vi "Port.vi"(8 "error in (no error)":errorcluster, 11 "Node Ptr":T1 format="%.0x") -> (0 "error out":errorcluster)   [LabVIEW 2020, in "Communication Bus Template System Explorer.lvlib" / "Implementation.lvlib"]
uses:
  Implementation.lvlib
  <vilib>/NI VeriStand/Custom Device API/Custom Device Item Ref.ctl
  <vilib>/NI VeriStand/Custom Device API/Custom Device API.lvlib
  Scripting/Communication Bus Template Scripting.lvlib
panel:
  in  "Baud Rate":u32
  in  "Database":string(combo)
  in  "SHDocVw.IWebBrowser":refnum<k7>(container)
  in  "Specific Header":cluster{"Section Name":string}={"Section Name"="Specific Page Settings"}
  in  "General Header":cluster{"Section Name":string}={"Section Name"="General Page Settings"}
  in  "Description":string
  in  "Name":string
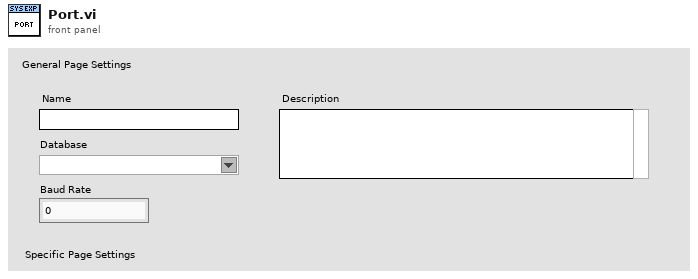
[diagram p1: front panel]
types:
  T1 = typedef "Custom Device API.lvlib/Custom Device Item Ref.ctl" = u64
  T2 = typedef "Custom Device API.lvlib/Custom Device Item Info.ctl" = cluster{"Name":string, "Is Channel":bool, "GUID":string, "Is Waveform":bool}
  T3 = typedef "Custom Device API.lvlib/Custom Device Commands.ctl" = enum16{"Default", "Item renamed", "Shutdown", "Dynamic button pressed"}
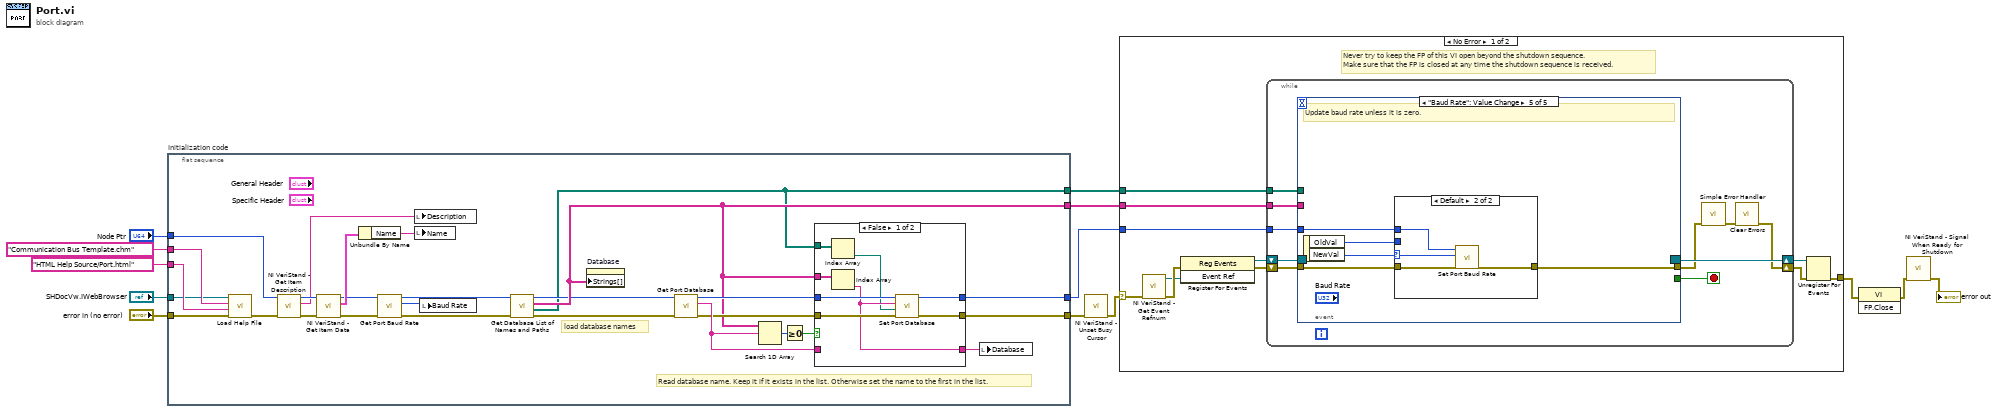
[diagram p0: block diagram]
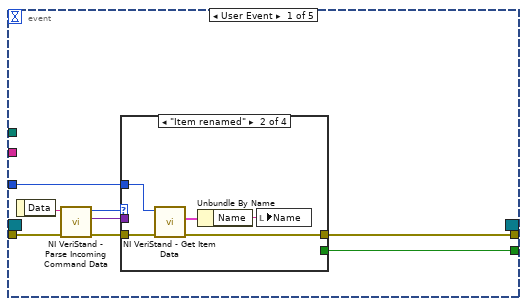
[diagram p3: hidden frame]
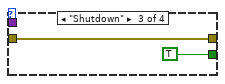
[diagram p5: hidden frame]
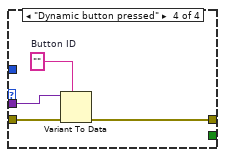
[diagram p6: hidden frame]
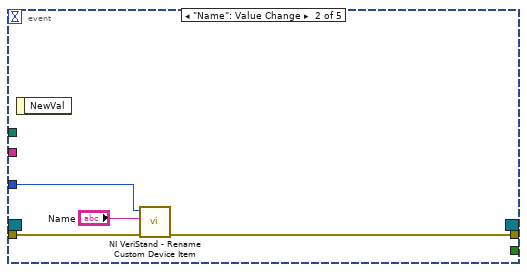
[diagram p7: hidden frame]
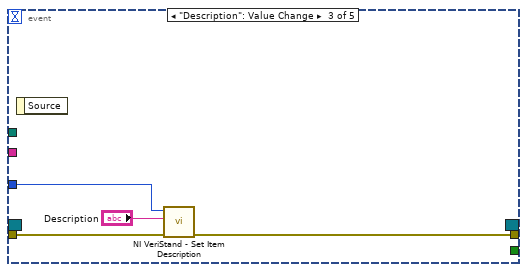
[diagram p8: hidden frame]
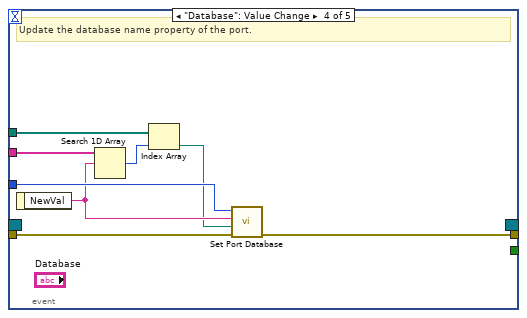
[diagram p9: hidden frame]
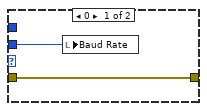
[diagram p10: hidden frame]
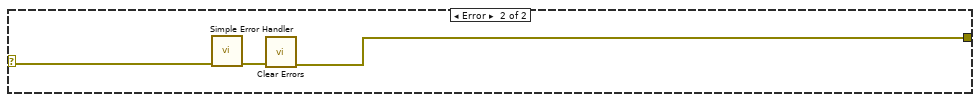
[diagram p11: hidden frame]
diagram:
  n1 = flat-sequence "Initialization code" {
    tunnel: "error in (no error)" -> [w35]
    tunnel: "Node Ptr" -> [w38]
    tunnel: [w30] -> w9
    tunnel: [w29] -> w6
    tunnel: "SHDocVw.IWebBrowser" -> [w31]
    tunnel: "HTML Help Source/Port.html" ("CD_CHM_Section") -> [w33]
    tunnel: "Communication Bus Template.chm" ("CD_CHM_FileName") -> [w32]
    tunnel: [w14] -> w2
    tunnel: [w18] -> w1
    frame #0 {
      # "Read database name. Keep it if it exists in the list. Otherwise set the name to the first in the list."
      # "load database names"
      n2 = call "Load Help File.vi"("error in (no error)"=w35, "HTML File to Load"=w33, "Main CHM File"=w32, "Browser"=w31) -> ("error out"=w34:errorcluster)  [unwired: 7 in]
      n3 = call <vilib>:"NI VeriStand - Get Item Description.vi"("error in (no error)"=w34, "Item Ref in"=w38) -> ("error out"=w40:errorcluster, "Description"=w36:string, "Item Ref out"=w41:T1)  [unwired: 7 out]
      n4 = call <vilib>:"NI VeriStand - Get Item Data.vi"("error in (no error)"=w40, "Item Ref in"=w41) -> ("error out"=w22:errorcluster, "Item Info"=w39:T2, "Item Ref out"=w21:T1)  [unwired: 7 out]
      n5 = Unbundle By Name(w39) -> ("Name"=w37:string)
      n6 = call "Get Port Baud Rate.vi"("error in"=w22, "Port Ref"=w21) -> ("error out"=w19:errorcluster, "Baud Rate"=w23:u32, "Port Ref out"=w20:T1)  [unwired: 7 in]
      n7 = local write "Description"(w36) -> ()
      n8 = local write "Name"(w37) -> ()
      n9 = local write "Baud Rate"(w23) -> ()
      n10 = call "Get Database List of Names and Paths.vi"("error in"=w19, "Databases section Ref"=w20) -> ("error out"=w16:errorcluster, "Paths"=w14:path[], "Names"=w18:string[], "Databases section Ref out"=w17:T1)  [unwired: 6 in]
      n11 = property on="Database" class="CmbBox"("Strings[]"=w18) -> ()  [unwired: 2 in, 2 out]
      n12 = call "Get Port Database.vi"("error in"=w16, "Port Ref"=w17) -> ("error out"=w24:errorcluster, "Database Name"=w25:string, "Port Ref out"=w28:T1)  [unwired: 5 in, 2 out]
      n13 = Search 1D Array(1D array=w18, element=w25) -> (index of element=w15:i32)  [unwired: 1 in]
      n14 = Greater Or Equal To 0?(x=w15) -> (x >= 0?=w27:bool)
      n15 = case shown="False" w27 {
        tunnel: [w46 w51] -> w30
        tunnel: [w47 w52] -> w29
        tunnel: w24 -> [w45 w51]
        tunnel: w28 -> [w48 w52]
        tunnel: [w44 w50] -> w26
        tunnel: w25 -> [_ w50]
        tunnel: w18 -> [w49 _]
        tunnel: w14 -> [w43 _]
        frame False {
          n16 = Index Array(array=w43) -> (element=w42:path)  [unwired: 1 in]
          n17 = Index Array(array=w49) -> (element=w44:string)  [unwired: 1 in]
          n18 = call "Set Port Database.vi"("error in"=w45, "Database Path"=w42, "Database Name"=w44, "Port Ref"=w48) -> ("error out"=w46:errorcluster, "Port Ref out"=w47:T1)  [unwired: 6 in]
        }
        frame True {
        }
      }
      n19 = local write "Database"(w26) -> ()
    }
  }
  n20 = call <vilib>:"NI VeriStand - Unset Busy Cursor.vi"("error in (no error)"=w9) -> ("error out"=w8:errorcluster)  [unwired: 10 out]
  n21 = case shown="No Error" w8 {
    selector: w8 -> [w55 w123]
    tunnel: [w60 w121] -> w13
    tunnel: w6 -> [w56 _]
    tunnel: w2 -> [w54 _]
    tunnel: w1 -> [w53 _]
    frame No Error {
      # "Never try to keep the FP of this VI open beyond the shutdown sequence.\nMake sure that the FP is closed at any time the shutdown sequence is received."
      n22 = call <vilib>:"NI VeriStand - Get Event Refnum.vi"("error in (no error)"=w55) -> ("error out"=w63:errorcluster, "Event Ref"=w59:refnum<user-event>)  [unwired: 9 out]
      n23 = register-events(error in=w63, w59) -> (reference out=w57:refnum<event-registration>, error out=w58:errorcluster)  [unwired: 1 in]
      n24 = while {
        tunnel: w56 -> [w69]
        shift-right: [w66] -> w61
        shift-left: w58 -> [w72]
        shift-right: [w73] -> w62
        shift-left: w57 -> [w71]
        tunnel: w54 -> [w65]
        tunnel: w53 -> [w64]
        stop <- w70 stop-if-true
        n25 = event shown="[4] \"Baud Rate\": Value Change" {
          selector: w71 -> [_ _ _ _ _]
          dyn-events: [_ _ _ _ _] -> w73
          timeout: _ -> [_ _ _ _ _]
          tunnel: w72 -> [w81 w97 w100 w109 w114]
          tunnel: [w77 _ _ _ _] -> w70
          tunnel: [w76 w96 w99 w105 w112] -> w68
          tunnel: w69 -> [w75 w95 w101 w104 w111]
          tunnel: w65 -> [_ _ _ w108 _]
          tunnel: w64 -> [_ _ _ w107 _]
          event User Event {
            n26 = event-data() -> ("Data"=w80:string)  [unwired: 1 out]
            n27 = call <vilib>:"NI VeriStand - Parse Incoming Command Data.vi"("error in (no error)"=w81, "Incoming data"=w80) -> ("error out"=w79:errorcluster, "Outgoing data"=w74:variant, "Action"=w78:T3)  [unwired: 7 out]
            n28 = case shown="\"Item renamed\"" w78 {
              tunnel: w79 -> [w82 w87 w88 w93]
              tunnel: [_ _ TRUE _] -> w77
              tunnel: [w82 w84 w88 w90] -> w76
              tunnel: w75 -> [_ w86 _ _]
              tunnel: w74 -> [_ _ _ w92]
              frame "Default", Default {
              }
              frame "Item renamed" {
                n29 = call <vilib>:"NI VeriStand - Get Item Data.vi"("error in (no error)"=w87, "Item Ref in"=w86) -> ("error out"=w84:errorcluster, "Item Info"=w85:T2)  [unwired: 8 out]
                n30 = Unbundle By Name(w85) -> ("Name"=w83:string)
                n31 = local write "Name"(w83) -> ()
              }
              frame "Shutdown" {
              }
              frame "Dynamic button pressed" {
                w91 = ""  # Button ID
                n32 = Variant To Data(error in=w93, type=w91, Variant=w92) -> (error out=w90:errorcluster)  [unwired: 1 out]
              }
            }
          }
          event "Name": Value Change {
            n33 = event-data() -> ()  [unwired: 2 out]
            n34 = call <vilib>:"NI VeriStand - Rename Custom Device Item.vi"("error in (no error)"=w97, "New Name"="Name", "Item Ref in"=w95) -> ("error out"=w96:errorcluster)  [unwired: 1 in, 7 out]
          }
          event "Description": Value Change {
            n35 = event-data() -> ()  [unwired: 2 out]
            n36 = call <vilib>:"NI VeriStand - Set Item Description.vi"("error in (no error)"=w100, "Description"="Description", "Item Ref in"=w101) -> ("error out"=w99:errorcluster)  [unwired: 8 out]
          }
          event "Database": Value Change {
            # "Update the database name property of the port."
            n37 = event-data() -> ("NewVal"=w103:string)  [unwired: 1 out]
            n38 = Search 1D Array(1D array=w107, element=w103) -> (index of element=w106:i32)  [unwired: 1 in]
            n39 = Index Array(array=w108, index=w106) -> (element=w102:path)
            n40 = call "Set Port Database.vi"("error in"=w109, "Database Path"=w102, "Database Name"=w103, "Port Ref"=w104) -> ("error out"=w105:errorcluster)  [unwired: 6 in, 1 out]
          }
          event "Baud Rate": Value Change {
            # "Update baud rate unless it is zero."
            n41 = event-data() -> ("OldVal"=w110:u32, "NewVal"=w113:u32)  [unwired: 1 out]
            n42 = case shown="Default" w113 {
              selector: w113 -> [_ w117]
              tunnel: w114 -> [w116 w120]
              tunnel: [w116 w119] -> w112
              tunnel: w111 -> [_ w118]
              tunnel: w110 -> [w115 _]
              frame 0 {
                n43 = local write "Baud Rate"(w115) -> ()
              }
              frame Default {
                n44 = call "Set Port Baud Rate.vi"("error in"=w120, "Baud Rate"=w117, "Port Ref"=w118) -> ("error out"=w119:errorcluster)  [unwired: 7 in, 1 out]
              }
            }
          }
        }
        n45 = call <vilib>:"Simple Error Handler.vi"("error in (no error)"=w68) -> ("error out"=w67:errorcluster)  [unwired: 1 in, 7 out]
        n46 = call <vilib>:"Clear Errors.vi"("error in (no error)"=w67) -> ("error out"=w66:errorcluster)  [unwired: 1 in, 5 out]
      }
      n47 = Unregister For Events(event registration refnum=w62, error in=w61) -> (error out=w60:errorcluster)
    }
    frame Error {
      n48 = call <vilib>:"Simple Error Handler.vi"("error in (no error)"=w123) -> ("error out"=w122:errorcluster)  [unwired: 1 in, 7 out]
      n49 = call <vilib>:"Clear Errors.vi"("error in (no error)"=w122) -> ("error out"=w121:errorcluster)  [unwired: 1 in, 5 out]
    }
  }
  n50 = invoke class="VI" method="FP.Close"(error in=w13) -> (error out=w12:errorcluster)  [unwired: 2 in, 2 out]
  n51 = call <vilib>:"NI VeriStand - Signal When Ready for Shutdown.vi"("error in (no error)"=w12) -> ("error out"=→"error out":errorcluster)  [unwired: 10 out]
